vi "Configure Accelerometer SPI.vi"(5 "gyro range (deg/sec)":u16(ring)=250 items=["250"=250, "500"=500, "1000"=1000, "2000"=2000], 7 "accel range (g)":u16(ring)=2 items=["2"=2, "4"=4, "8"=8, "16"=16], 8 "error in (no error)":errorcluster, 11 "Accelerometer":T1) -> (0 "error out":errorcluster, 3 "Accelerometer out":T1)   [LabVIEW 2013]
doc: "Use this template to build a VI to use as a subVI."
uses:
  AccelerometerSPI.ctl
  <vilib>/ni845x/ni845x.llb/ni845xControl.ctl
  <vilib>/ni845x/ni845x.llb/ni845xSpiConfiguration.ctl
  9250registers.ctl
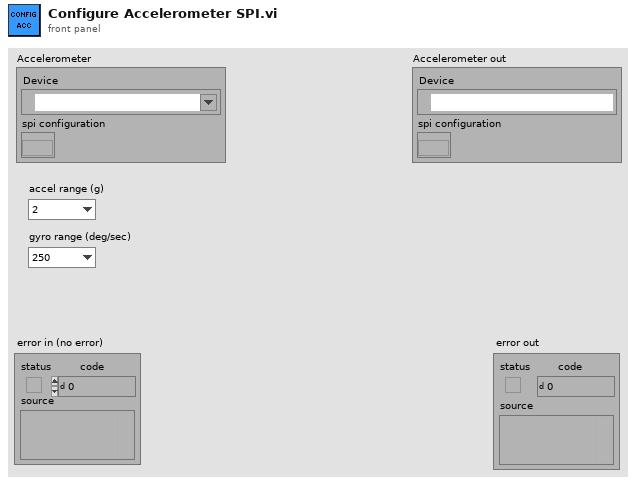
[diagram p1: front panel]
types:
  T1 = typedef "AccelerometerSPI.ctl" = cluster{"Device":T2, "spi configuration":T3}
  T2 = typedef "ni845xControl.ctl" = refnum<k21>
  T3 = typedef "ni845xSpiConfiguration.ctl" = refnum<k20>
  T4 = typedef "9250registers.ctl" = u8
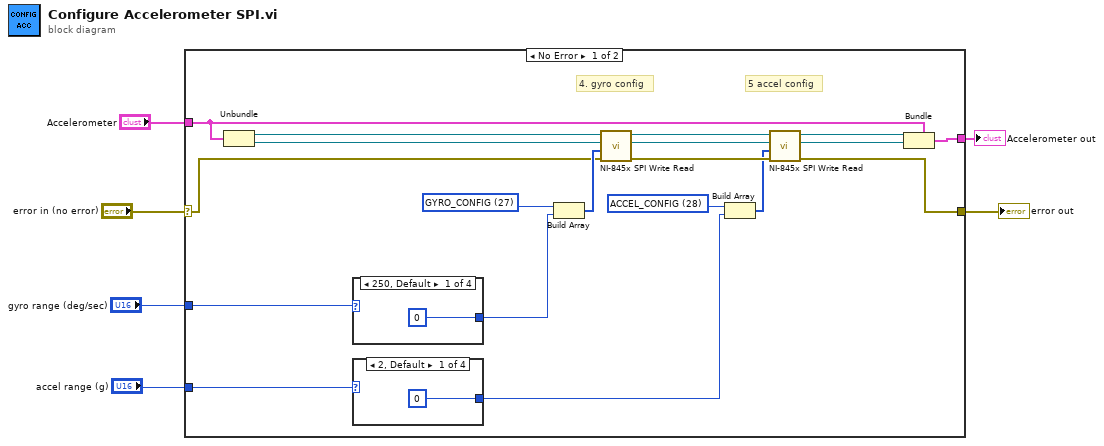
[diagram p0: block diagram]
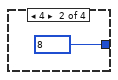
[diagram p2: hidden frame]
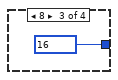
[diagram p3: hidden frame]
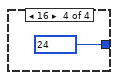
[diagram p4: hidden frame]
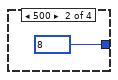
[diagram p5: hidden frame]
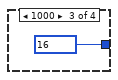
[diagram p6: hidden frame]
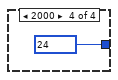
[diagram p7: hidden frame]
diagram:
  n1 = case shown="No Error" "error in (no error)" {
    selector: "error in (no error)" -> [w7 w35]
    tunnel: [w10 w35] -> w5
    tunnel: "Accelerometer" -> [w25 w34]
    tunnel: [w24 w34] -> w3
    tunnel: "gyro range (deg/sec)" -> [w23 _]
    tunnel: "accel range (g)" -> [w20 _]
    frame No Error {
      w19 = T4 28 items=["SELF_TEST_X_GYRO"=0, "SELF_TEST_Y_GYRO"=1, "SELF_TEST_Z_GYRO"=2, "SELF_TEST_X_ACCEL"=13, "SELF_TEST_Y_ACCEL"=14, "SELF_TEST_Z_ACCEL"=15, "XG_OFFSET"=19, "YG_OFFSET"=21, "ZG_OFFSET"=23, "SMPLRT_DIV"=25, "CONFIG"=26, "GYRO_CONFIG"=27, "ACCEL_CONFIG"=28, "ACCEL_CONFIG2"=29, "FIFO_EN"=35, "I2C_MST_CTRL"=36, "I2C_SLV0_ADDR"=37, "I2C_SLV0_REG"=38, "I2C_SLV0_CTRL"=39, "I2C_MST_STATUS"=54, "INT_ENABLE"=56, "INT_STATUS"=58, "ACCEL_XOUT"=59, "ACCEL_YOUT"=61, "ACCEL_ZOUT"=63, "TEMP_OUT"=65, "GYRO_XOUT"=67, "GYRO_YOUT"=69, "GYRO_ZOUT"=71, "EXT_SENS_DATA_00"=73, "I2C_SLV0_D0"=99, "USER_CTRL"=106, "PWR_MGMT_1"=107, "PWR_MGMT_2"=108, "WHO_AM_I"=117, "XA_OFFSET"=119, "YA_OFFSET"=122, "ZA_OFFSET"=125]
      w22 = T4 27 items=["SELF_TEST_X_GYRO"=0, "SELF_TEST_Y_GYRO"=1, "SELF_TEST_Z_GYRO"=2, "SELF_TEST_X_ACCEL"=13, "SELF_TEST_Y_ACCEL"=14, "SELF_TEST_Z_ACCEL"=15, "XG_OFFSET"=19, "YG_OFFSET"=21, "ZG_OFFSET"=23, "SMPLRT_DIV"=25, "CONFIG"=26, "GYRO_CONFIG"=27, "ACCEL_CONFIG"=28, "ACCEL_CONFIG2"=29, "FIFO_EN"=35, "I2C_MST_CTRL"=36, "I2C_SLV0_ADDR"=37, "I2C_SLV0_REG"=38, "I2C_SLV0_CTRL"=39, "I2C_MST_STATUS"=54, "INT_ENABLE"=56, "INT_STATUS"=58, "ACCEL_XOUT"=59, "ACCEL_YOUT"=61, "ACCEL_ZOUT"=63, "TEMP_OUT"=65, "GYRO_XOUT"=67, "GYRO_YOUT"=69, "GYRO_ZOUT"=71, "EXT_SENS_DATA_00"=73, "I2C_SLV0_D0"=99, "USER_CTRL"=106, "PWR_MGMT_1"=107, "PWR_MGMT_2"=108, "WHO_AM_I"=117, "XA_OFFSET"=119, "YA_OFFSET"=122, "ZA_OFFSET"=125]
      # "5 accel config"
      # "4. gyro config"
      n2 = Unbundle(w25) -> ("Device"=w9:T2, "spi configuration"=w8:T3)
      n3 = case shown="250, Default" w23 {
        tunnel: [u8 0 u8 8 u8 16 u8 24] -> w21
        frame 250, Default {
        }
        frame 500 {
        }
        frame 1000 {
        }
        frame 2000 {
        }
      }
      n4 = case shown="2, Default" w20 {
        tunnel: [u8 0 u8 8 u8 16 u8 24] -> w18
        frame 2, Default {
        }
        frame 4 {
        }
        frame 8 {
        }
        frame 16 {
        }
      }
      n5 = Build Array(w22, w21) -> (w17:T4[])
      n6 = call <vilib>:"NI-845x SPI Write Read.vi"("error in (no error)"=w7, "write data"=w17, "spi configuration in"=w8, "device reference in"=w9) -> ("error out"=w14:errorcluster, "spi configuration out"=w15:T3, "device reference out"=w16:T2)  [unwired: 4 in, 1 out]
      n7 = Build Array(w19, w18) -> (w13:T4[])
      n8 = call <vilib>:"NI-845x SPI Write Read.vi"("error in (no error)"=w14, "write data"=w13, "spi configuration in"=w15, "device reference in"=w16) -> ("error out"=w10:errorcluster, "spi configuration out"=w11:T3, "device reference out"=w12:T2)  [unwired: 4 in, 1 out]
      n9 = Bundle(cluster=w25, "Device"=w12, "spi configuration"=w11) -> (w24:T1)
    }
    frame Error {
    }
  }
  "error out" <- w5
  "Accelerometer out" <- w3
